vi "CSS grouping with vector space.vi"() -> ()   [LabVIEW 2014]
uses:
  <vilib>/Utility/file.llb/Read From Spreadsheet File (string).vi
  <vilib>/Utility/file.llb/Write To Spreadsheet File (string).vi
panel:
  in  "file path (to write) 2":path
  in  "save":bool
  in  "cycles":i32=1
  out "Array 4":string[](array[string])
  in  "cluster centers (original) 7":string[](array[string])=["0 -1 1 -4 0", "0 -1 2 -2 0", "0 -2 3 -3 0", "0 -3 4 -4 0", "0 -1 1 -4 4 -3 0", "0 -1 2 -2 3 -3 0", "0 -4 1 -1 2 -2 0", "0 -4 4 -3 3 -2 0", "0 -1 1 -4 0 -2 3 -3 0", "0 -1 2 -2 0 -4 4 -3 0"]
  out "vector positions only":dbl[][](array[numeric])
  out "Array 3":dbl[][](array[numeric])
  out "Array 2":dbl[][](array[numeric])
  out "Array":dbl[][](array[numeric])
  out "Assignment (enhanced)":string[](array[string])
  out "Assignment":string[](array[string])
  out "all rows":string[][](array[string])
  in  "cluster centers (original) 5":string[](array[string])=["0 -1 1 -4 0 -4 1 -1 0 -1 1 -4 0 -4 1 -1 0 -1 1 -4 0 -4 1 -1 0 -1 0 -1 1 -4 0 -4 1 -1 0", "0 -1 2 -2 0 -2 2 -1 0 -1 2 -2 0 -2 2 -1 0 -1 2 -2 0 -2 2 -1 0 -1 0 -1 2 -2 0 -2 2 -1 0", "0 -2 3 -3 0 -3 3 -2 0 -2 3 -3 0 -3 3 -2 0 -2 3 -3 0 -3 3 -2 0 -2 0 -2 3 -3 0 -3 3 -2 0", "0 -3 4 -4 0 -4 4 -3 0 -3 4 -4 0 -4 4 -3 0 -3 4 -4 0 -4 4 -3 0 -3 0 -3 4 -4 0 -4 4 -3 0", "0 -1 1 -4 4 -3 0 -3 4 -4 1 -1 0 -1 1 -4 4 -3 0 -3 4 -4 1 -1 0 -1 1 -4 4 -3 0 -3 4 -4 1 -1 0 -1 1 -4 4 -3 0 -3 4 -4 1 -1 0", "0 -1 2 -2 3 -3 0 -3 3 -2 2 -1 0 -1 2 -2 3 -3 0 -3 3 -2 2 -1 0 -1 2 -2 3 -3 0 -3 3 -2 2 -1 0 -1 2 -2 3 -3 0 -3 3 -2 2 -1 0", "0 -4 1 -1 2 -2 0 -2 2 -1 1 -4 0 -4 1 -1 2 -2 0 -2 2 -1 1 -4 0 -4 1 -1 2 -2 0 -2 2 -1 1 -4 0 -4 1 -1 2 -2 0 -2 2 -1 1 -4 0", "0 -4 4 -3 3 -2 0 -2 3 -3 4 -4 0 -4 4 -3 3 -2 0 -2 3 -3 4 -4 0 -4 4 -3 3 -2 0 -2 3 -3 4 -4 0 -4 4 -3 3 -2 0 -2 3 -3 4 -4 0", "0 -1 1 -4 0 -2 3 -3 0 -3 3 -2 0 -4 1 -1 0 -1 1 -4 0 -2 3 -3 0 -3 3 -2 0 -4 1 -1 0 -1 1 -4 0 -2 3 -3 0 -3 3 -2 0 -4 1 -1 0 -1 1 -4 0 -2 3 -3 0 -3 3 -2 0 -4 1 -1 0", "0 -1 2 -2 0 -4 4 -3 0 -3 4 -4 0 -2 2 -1 0 -1 2 -2 0 -4 4 -3 0 -3 4 -4 0 -2 2 -1 0 -1 2 -2 0 -4 4 -3 0 -3 4 -4 0 -2 2 -1 0 -1 2 -2 0 -4 4 -3 0 -3 4 -4 0 -2 2 -1 0"]
  in  "cluster centers (original) 4":string[](array[string])=["0 -1 1 -4 0 -4 1 -1 0 -1 1 -4 0 -4 1 -1 0", "0 -1 2 -2 0 -2 2 -1 0 -1 2 -2 0 -2 2 -1 0", "0 -2 3 -3 0 -3 3 -2 0 -2 3 -3 0 -3 3 -2 0", "0 -3 4 -4 0 -4 4 -3 0 -3 4 -4 0 -4 4 -3 0", "0 -1 1 -4 4 -3 0 -3 4 -4 1 -1 0 -1 1 -4 4 -3 0 -3 4 -4 1 -1 0", "0 -1 2 -2 3 -3 0 -3 3 -2 2 -1 0 -1 2 -2 3 -3 0 -3 3 -2 2 -1 0", "0 -4 1 -1 2 -2 0 -2 2 -1 1 -4 0 -4 1 -1 2 -2 0 -2 2 -1 1 -4 0", "0 -4 4 -3 3 -2 0 -2 3 -3 4 -4 0 -4 4 -3 3 -2 0 -2 3 -3 4 -4 0", "0 -1 1 -4 0 -2 3 -3 0 -3 3 -2 0 -4 1 -1 0 -1 1 -4 0 -2 3 -3 0 -3 3 -2 0 -4 1 -1 0", "0 -1 2 -2 0 -4 4 -3 0 -3 4 -4 0 -2 2 -1 0 -1 2 -2 0 -4 4 -3 0 -3 4 -4 0 -2 2 -1 0"]
  out "size(s)":i32
  in  "cluster centers (original) 3":string[](array[string])=["0 -1 1 -4 0 -4 1 -1 0 -1 1 -4 0 -4 1 -1 0 -1 1 -4 0 -4 1 -1 0", "0 -1 2 -2 0 -2 2 -1 0 -1 2 -2 0 -2 2 -1 0 -1 2 -2 0 -2 2 -1 0", "0 -2 3 -3 0 -3 3 -2 0 -2 3 -3 0 -3 3 -2 0 -2 3 -3 0 -3 3 -2 0", "0 -3 4 -4 0 -4 4 -3 0 -3 4 -4 0 -4 4 -3 0 -3 4 -4 0 -4 4 -3 0", "0 -1 1 -4 4 -3 0 -3 4 -4 1 -1 0 -1 1 -4 4 -3 0 -3 4 -4 1 -1 0 -1 1 -4 4 -3 0 -3 4 -4 1 -1 0", "0 -1 2 -2 3 -3 0 -3 3 -2 2 -1 0 -1 2 -2 3 -3 0 -3 3 -2 2 -1 0 -1 2 -2 3 -3 0 -3 3 -2 2 -1 0", "0 -4 1 -1 2 -2 0 -2 2 -1 1 -4 0 -4 1 -1 2 -2 0 -2 2 -1 1 -4 0 -4 1 -1 2 -2 0 -2 2 -1 1 -4 0", "0 -4 4 -3 3 -2 0 -2 3 -3 4 -4 0 -4 4 -3 3 -2 0 -2 3 -3 4 -4 0 -4 4 -3 3 -2 0 -2 3 -3 4 -4 0", "0 -1 1 -4 0 -2 3 -3 0 -3 3 -2 0 -4 1 -1 0 -1 1 -4 0 -2 3 -3 0 -3 3 -2 0 -4 1 -1 0 -1 1 -4 0 -2 3 -3 0 -3 3 -2 0 -4 1 -1 0", "0 -1 2 -2 0 -4 4 -3 0 -3 4 -4 0 -2 2 -1 0 -1 2 -2 0 -4 4 -3 0 -3 4 -4 0 -2 2 -1 0 -1 2 -2 0 -4 4 -3 0 -3 4 -4 0 -2 2 -1 0"]
  in  "cluster centers (original) 2":string[](array[string])=["0 -1 1 -4 0 -4 1 -1 0", "0 -1 2 -2 0 -2 2 -1 0", "0 -2 3 -3 0 -3 3 -2 0", "0 -3 4 -4 0 -4 4 -3 0", "0 -1 1 -4 4 -3 0 -3 4 -4 1 -1 0", "0 -1 2 -2 3 -3 0 -3 3 -2 2 -1 0", "0 -4 1 -1 2 -2 0 -2 2 -1 1 -4 0", "0 -4 4 -3 3 -2 0 -2 3 -3 4 -4 0", "0 -1 1 -4 0 -2 3 -3 0 -3 3 -2 0 -4 1 -1 0", "0 -1 2 -2 0 -4 4 -3 0 -3 4 -4 0 -2 2 -1 0"]
  out "accuracy":string[][](array[string])
  in  "cluster centers (original) long 5":string[](array[string])=["1 0 -1 1 -1 0 -4 1 -4 0 1 0 -1 1 -1 0 -4 1 -4 0 1 0 -1 1 -1 0 -4 1 -4 0 1 0 -1 1 -1 0 -4 1 -4 0 1 0 -1 1 -1 0 -4 1 -4 0 1", "2 0 -1 2 -1 0 -2 2 -2 0 2 0 -1 2 -1 0 -2 2 -2 0 2 0 -1 2 -1 0 -2 2 -2 0 2 0 -1 2 -1 0 -2 2 -2 0 2 0 -1 2 -1 0 -2 2 -2 0 2", "3 0 -3 3 -3 0 -2 3 -2 0 3 0 -3 3 -3 0 -2 3 -2 0 3 0 -3 3 -3 0 -2 3 -2 0 3 0 -3 3 -3 0 -2 3 -2 0 3 0 -3 3 -3 0 -2 3 -2 0 3", "4 0 -3 4 -3 0 -4 4 -4 0 4 0 -3 4 -3 0 -4 4 -4 0 4 0 -3 4 -3 0 -4 4 -4 0 4 0 -3 4 -3 0 -4 4 -4 0 4 0 -3 4 -3 0 -4 4 -4 0 4", "-1 1 -4 0 -4 4 -3 4 -4 0 -4 1 -1 1 -4 0 -4 4 -3 4 -4 0 -4 1 -1 1 -4 0 -4 4 -3 4 -4 0 -4 1 -1 1 -4 0 -4 4 -3 4 -4 0 -4 1 -1 1 -4 0 -4 4 -3 4 -4 0 -4 1 -1", "-1 2 -2 0 -2 3 -3 3 -2 0 -2 2 -1 2 -2 0 -2 3 -3 3 -2 0 -2 2 -1 2 -2 0 -2 3 -3 3 -2 0 -2 2 -1 2 -2 0 -2 3 -3 3 -2 0 -2 2 -1 2 -2 0 -2 3 -3 3 -2 0 -2 2 -1", "-4 1 -1 0 -1 2 -2 2 -1 0 -1 1 -4 1 -1 0 -1 2 -2 2 -1 0 -1 1 -4 1 -1 0 -1 2 -2 2 -1 0 -1 1 -4 1 -1 0 -1 2 -2 2 -1 0 -1 1 -4 1 -1 0 -1 2 -2 2 -1 0 -1 1 -4", "-4 4 -3 0 -3 3 -2 3 -3 0 -3 4 -4 4 -3 0 -3 3 -2 3 -3 0 -3 4 -4 4 -3 0 -3 3 -2 3 -3 0 -3 4 -4 4 -3 0 -3 3 -2 3 -3 0 -3 4 -4 4 -3 0 -3 3 -2 3 -3 0 -3 4 -4", "0 -4 1 -1 0 -3 3 -2 3 -3 0 -1 1 -4 0 -4 1 -1 0 -3 3 -2 3 -3 0 -1 1 -4 0 -4 1 -1 0 -3 3 -2 3 -3 0 -1 1 -4 0 -4 1 -1 0 -3 3 -2 3 -3 0 -1 1 -4 0 -4 1 -1 0 -3 3 -2 3 -3 0 -1 1 -4 0", "0 -4 4 -3 0 -1 2 -2 2 -1 0 -3 4 -4 0 -4 4 -3 0 -1 2 -2 2 -1 0 -3 4 -4 0 -4 4 -3 0 -1 2 -2 2 -1 0 -3 4 -4 0 -4 4 -3 0 -1 2 -2 2 -1 0 -3 4 -4 0 -4 4 -3 0 -1 2 -2 2 -1 0 -3 4 -4 0"]
  in  "cluster centers (original) long 4":string[](array[string])=["1 0 -1 1 -1 0 -4 1 -4 0 1 0 -1 1 -1 0 -4 1 -4 0 1 0 -1 1 -1 0 -4 1 -4 0 1 0 -1 1 -1 0 -4 1 -4 0 1", "2 0 -1 2 -1 0 -2 2 -2 0 2 0 -1 2 -1 0 -2 2 -2 0 2 0 -1 2 -1 0 -2 2 -2 0 2 0 -1 2 -1 0 -2 2 -2 0 2", "3 0 -3 3 -3 0 -2 3 -2 0 3 0 -3 3 -3 0 -2 3 -2 0 3 0 -3 3 -3 0 -2 3 -2 0 3 0 -3 3 -3 0 -2 3 -2 0 3", "4 0 -3 4 -3 0 -4 4 -4 0 4 0 -3 4 -3 0 -4 4 -4 0 4 0 -3 4 -3 0 -4 4 -4 0 4 0 -3 4 -3 0 -4 4 -4 0 4", "-1 1 -4 0 -4 4 -3 4 -4 0 -4 1 -1 1 -4 0 -4 4 -3 4 -4 0 -4 1 -1 1 -4 0 -4 4 -3 4 -4 0 -4 1 -1 1 -4 0 -4 4 -3 4 -4 0 -4 1 -1", "-1 2 -2 0 -2 3 -3 3 -2 0 -2 2 -1 2 -2 0 -2 3 -3 3 -2 0 -2 2 -1 2 -2 0 -2 3 -3 3 -2 0 -2 2 -1 2 -2 0 -2 3 -3 3 -2 0 -2 2 -1", "-4 1 -1 0 -1 2 -2 2 -1 0 -1 1 -4 1 -1 0 -1 2 -2 2 -1 0 -1 1 -4 1 -1 0 -1 2 -2 2 -1 0 -1 1 -4 1 -1 0 -1 2 -2 2 -1 0 -1 1 -4", "-4 4 -3 0 -3 3 -2 3 -3 0 -3 4 -4 4 -3 0 -3 3 -2 3 -3 0 -3 4 -4 4 -3 0 -3 3 -2 3 -3 0 -3 4 -4 4 -3 0 -3 3 -2 3 -3 0 -3 4 -4", "0 -4 1 -1 0 -3 3 -2 3 -3 0 -1 1 -4 0 -4 1 -1 0 -3 3 -2 3 -3 0 -1 1 -4 0 -4 1 -1 0 -3 3 -2 3 -3 0 -1 1 -4 0 -4 1 -1 0 -3 3 -2 3 -3 0 -1 1 -4 0", "0 -4 4 -3 0 -1 2 -2 2 -1 0 -3 4 -4 0 -4 4 -3 0 -1 2 -2 2 -1 0 -3 4 -4 0 -4 4 -3 0 -1 2 -2 2 -1 0 -3 4 -4 0 -4 4 -3 0 -1 2 -2 2 -1 0 -3 4 -4 0"]
  in  "cluster centers (original) long 3":string[](array[string])=["1 0 -1 1 -1 0 -4 1 -4 0 1 0 -1 1 -1 0 -4 1 -4 0 1 0 -1 1 -1 0 -4 1 -4 0 1", "2 0 -1 2 -1 0 -2 2 -2 0 2 0 -1 2 -1 0 -2 2 -2 0 2 0 -1 2 -1 0 -2 2 -2 0 2", "3 0 -3 3 -3 0 -2 3 -2 0 3 0 -3 3 -3 0 -2 3 -2 0 3 0 -3 3 -3 0 -2 3 -2 0 3", "4 0 -3 4 -3 0 -4 4 -4 0 4 0 -3 4 -3 0 -4 4 -4 0 4 0 -3 4 -3 0 -4 4 -4 0 4", "-1 1 -4 0 -4 4 -3 4 -4 0 -4 1 -1 1 -4 0 -4 4 -3 4 -4 0 -4 1 -1 1 -4 0 -4 4 -3 4 -4 0 -4 1 -1", "-1 2 -2 0 -2 3 -3 3 -2 0 -2 2 -1 2 -2 0 -2 3 -3 3 -2 0 -2 2 -1 2 -2 0 -2 3 -3 3 -2 0 -2 2 -1", "-4 1 -1 0 -1 2 -2 2 -1 0 -1 1 -4 1 -1 0 -1 2 -2 2 -1 0 -1 1 -4 1 -1 0 -1 2 -2 2 -1 0 -1 1 -4", "-4 4 -3 0 -3 3 -2 3 -3 0 -3 4 -4 4 -3 0 -3 3 -2 3 -3 0 -3 4 -4 4 -3 0 -3 3 -2 3 -3 0 -3 4 -4", "0 -4 1 -1 0 -3 3 -2 3 -3 0 -1 1 -4 0 -4 1 -1 0 -3 3 -2 3 -3 0 -1 1 -4 0 -4 1 -1 0 -3 3 -2 3 -3 0 -1 1 -4 0", "0 -4 4 -3 0 -1 2 -2 2 -1 0 -3 4 -4 0 -4 4 -3 0 -1 2 -2 2 -1 0 -3 4 -4 0 -4 4 -3 0 -1 2 -2 2 -1 0 -3 4 -4 0"]
  in  "cluster centers (original) long":string[](array[string])=["1 0 -1 1 -1 0 -4 1 -4 0 1 0 -1 1 -1 0 -4 1 -4 0 1", "2 0 -1 2 -1 0 -2 2 -2 0 2 0 -1 2 -1 0 -2 2 -2 0 2", "3 0 -3 3 -3 0 -2 3 -2 0 3 0 -3 3 -3 0 -2 3 -2 0 3", "4 0 -3 4 -3 0 -4 4 -4 0 4 0 -3 4 -3 0 -4 4 -4 0 4", "-1 1 -4 0 -4 4 -3 4 -4 0 -4 1 -1 1 -4 0 -4 4 -3 4 -4 0 -4 1 -1", "-1 2 -2 0 -2 3 -3 3 -2 0 -2 2 -1 2 -2 0 -2 3 -3 3 -2 0 -2 2 -1", "-4 1 -1 0 -1 2 -2 2 -1 0 -1 1 -4 1 -1 0 -1 2 -2 2 -1 0 -1 1 -4", "-4 4 -3 0 -3 3 -2 3 -3 0 -3 4 -4 4 -3 0 -3 3 -2 3 -3 0 -3 4 -4", "0 -4 1 -1 0 -3 3 -2 3 -3 0 -1 1 -4 0 -4 1 -1 0 -3 3 -2 3 -3 0 -1 1 -4 0", "0 -4 4 -3 0 -1 2 -2 2 -1 0 -3 4 -4 0 -4 4 -3 0 -1 2 -2 2 -1 0 -3 4 -4 0"]
  out "Results":string[][](array[string])
  in  "file path (dialog if empty)":path=path "K:/PhD work/PhD research work 2/Common substring validation/documentation/Data final results/Common substrings (ground truth 2 CHECKED).txt"
  in  "cluster centers (original)":string[](array[string])=["1 0 -1 1 -1 0 -4 1 -4 0 1", "2 0 -1 2 -1 0 -2 2 -2 0 2", "3 0 -3 3 -3 0 -2 3 -2 0 3", "4 0 -3 4 -3 0 -4 4 -4 0 4", "-1 1 -4 0 -4 4 -3 4 -4 0 -4 1 -1", "-1 2 -2 0 -2 3 -3 3 -2 0 -2 2 -1", "-4 1 -1 0 -1 2 -2 2 -1 0 -1 1 -4", "-4 4 -3 0 -3 3 -2 3 -3 0 -3 4 -4", "0 -4 1 -1 0 -3 3 -2 3 -3 0 -1 1 -4 0", "0 -4 4 -3 0 -1 2 -2 2 -1 0 -3 4 -4 0"]
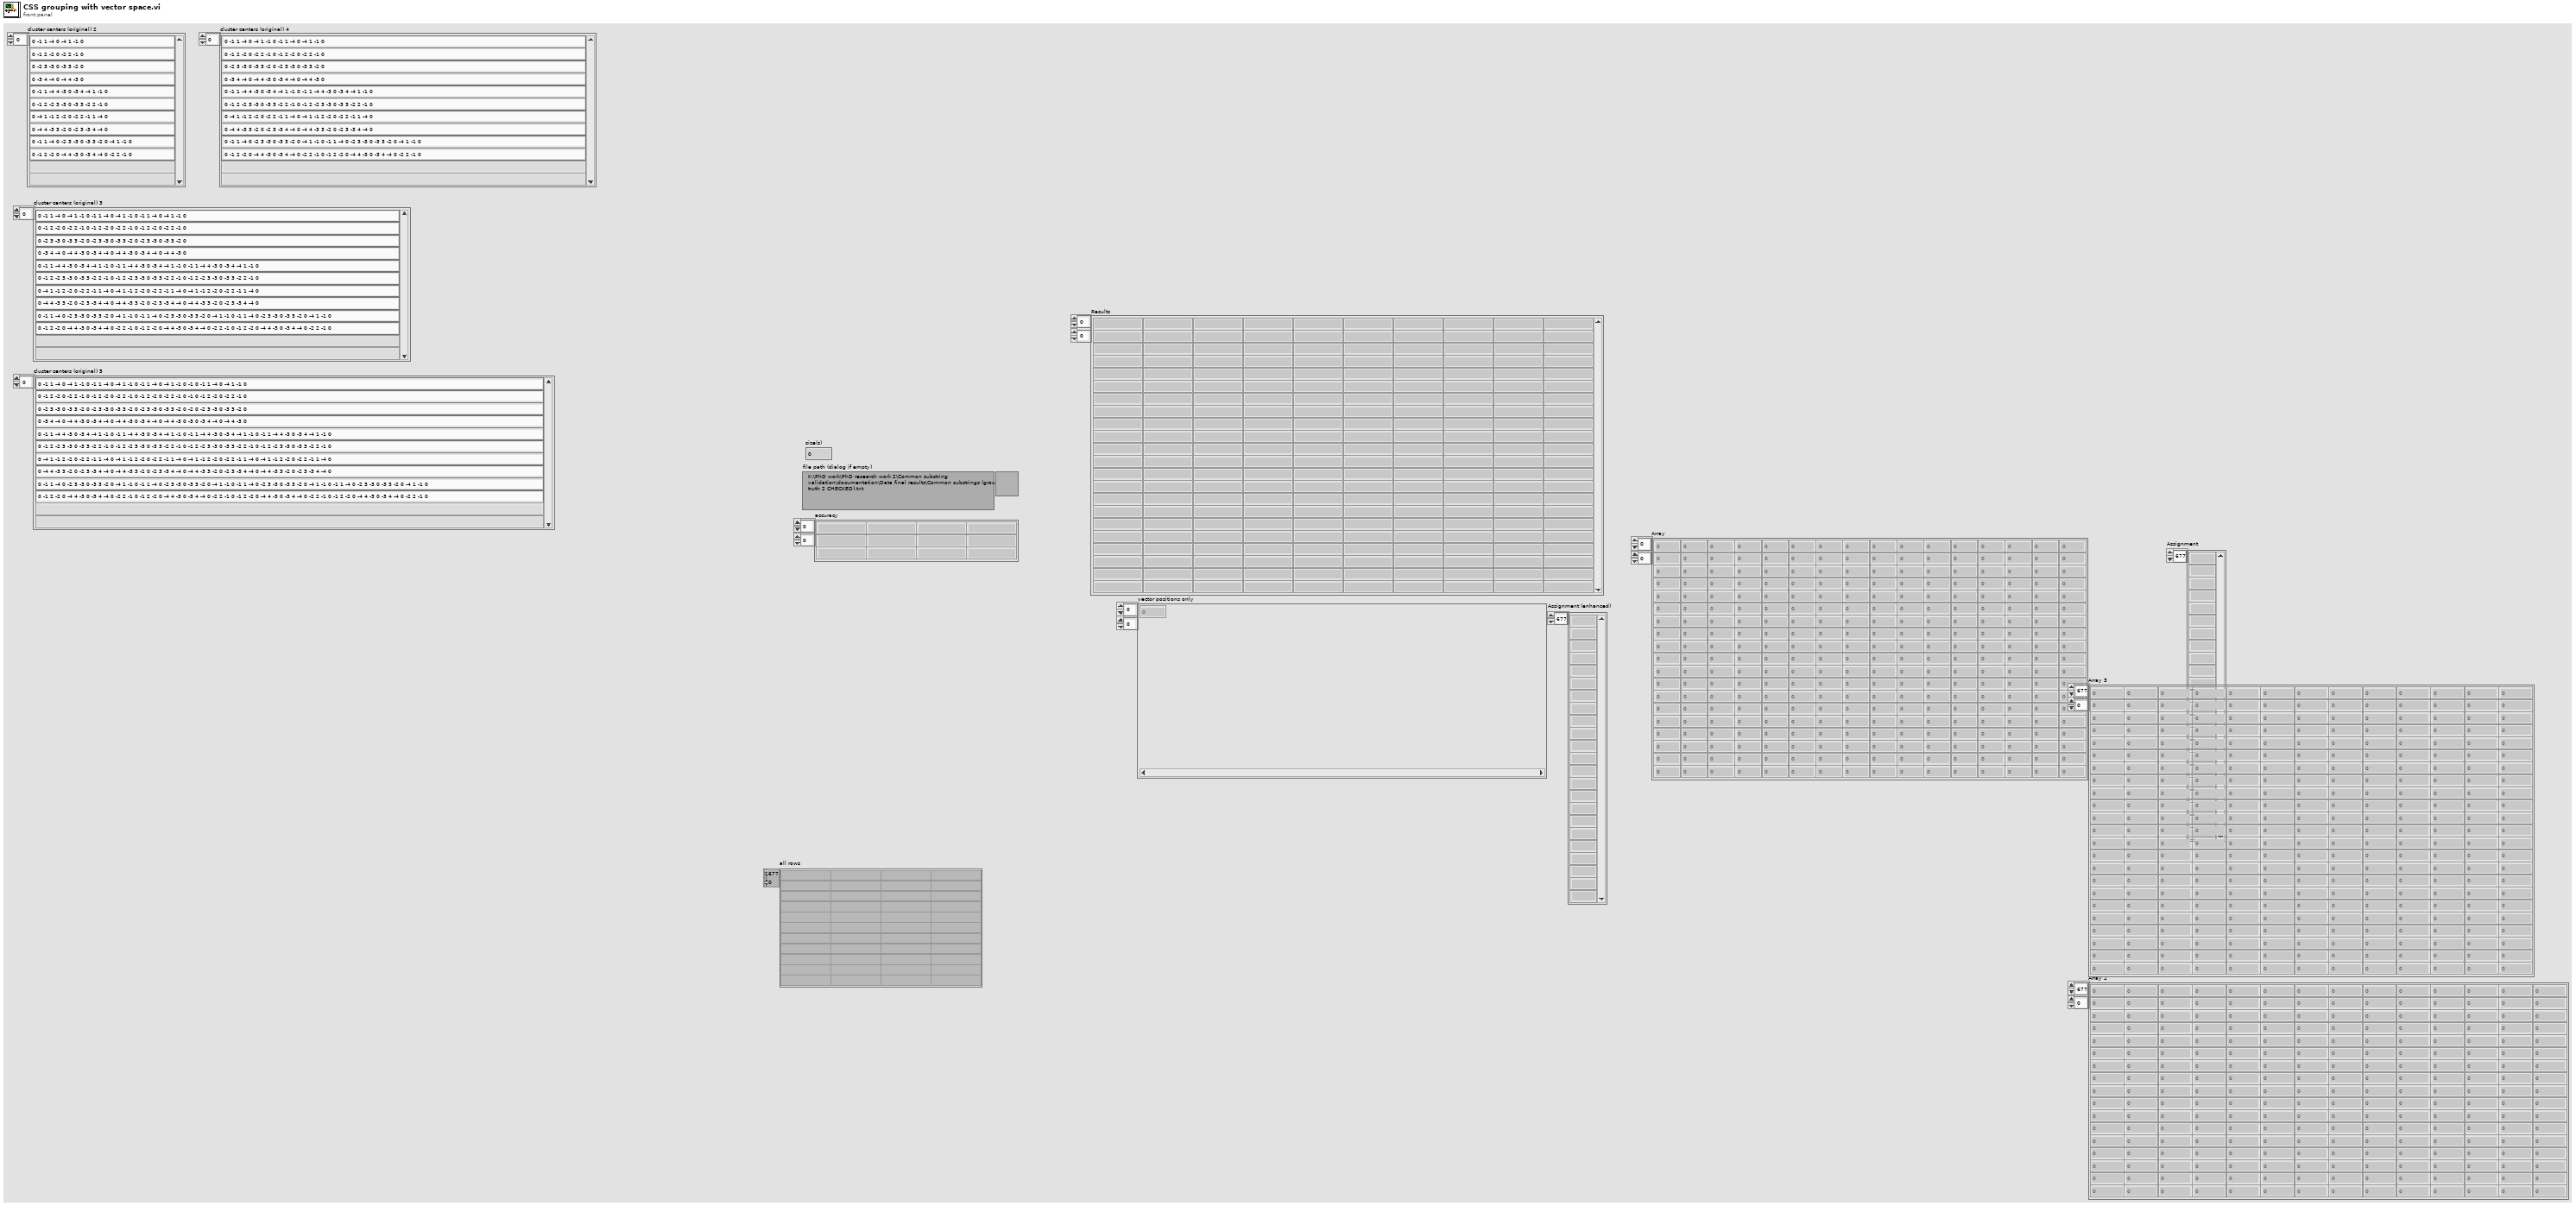
[diagram p1: front panel]
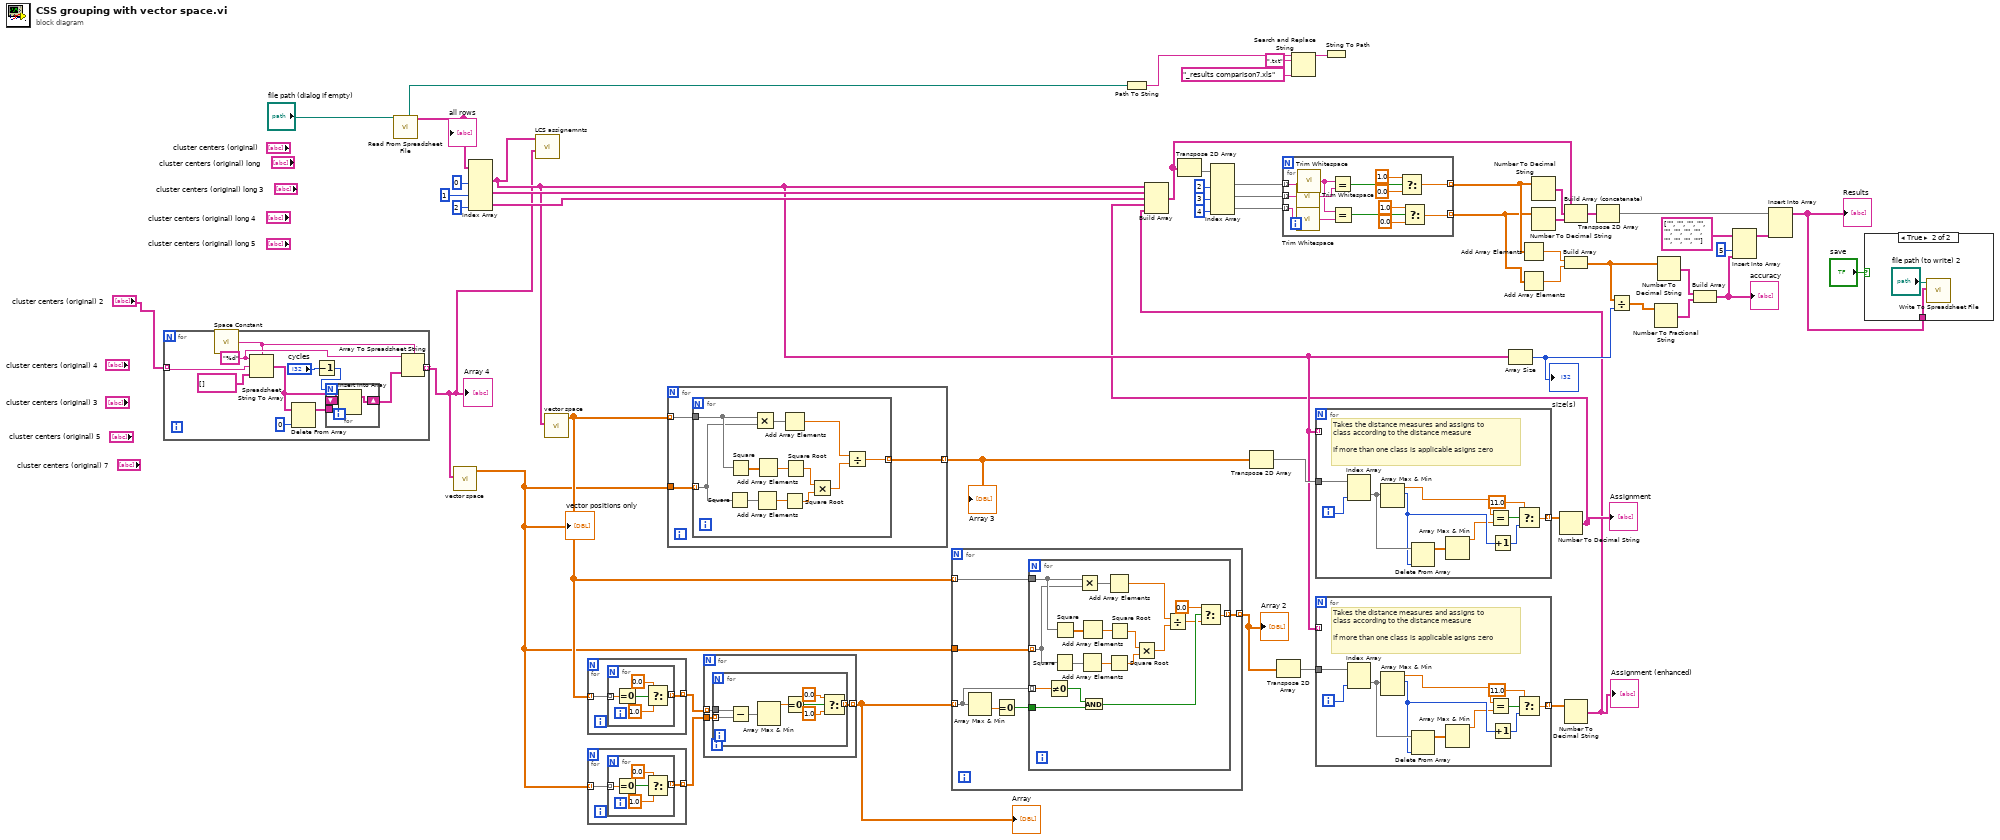
[diagram p0: block diagram]
diagram:
  n1 = for {
    tunnel: [w62] -> w4 mode=indexing
    tunnel: "cluster centers (original) 2" -> [w58] mode=indexing
    w63 = "%d" ("format string")
    n2 = call <vilib>:"Space Constant.vi"() -> ("String"=w61:string)
    n3 = Spreadsheet String To Array(delimiter (Tab)=w61, format string=w63, spreadsheet string=w58, array type (2D Dbl)=string[] []) -> (array=w57:string[])
    n4 = Delete From Array(array=w57, index=0) -> (array with subset deleted=w56:string[])  [unwired: 1 in, 1 out]
    n5 = Decrement(x="cycles") -> (x-1=w60:i32)
    n6 = for {
      N: w60 -> [_]
      tunnel: w56 -> [w68]
      shift-right: [w67] -> w64
      shift-left: w57 -> [w69]
      n7 = Insert Into Array(array=w69, new element=w68) -> (w67:string[])  [unwired: 1 in]
    }
    n8 = Array To Spreadsheet String(delimiter (Tab)=w61, array=w64, 3:w63) -> (spreadsheet string=w62:string)
  }
  "Array 4" <- w4
  n9 = call-poly <vilib>:"Read From Spreadsheet File.vi"("file path (dialog if empty)"="file path (dialog if empty)") -> ("all rows"=w21:string[][], "new file path (Not A Path if cancelled)"=w53:path)  [unwired: 6 in, 3 out]
  "all rows" <- w21
  n10 = call "vector space.vi"("Full transition sequence from service to end"=w4) -> ("vector positions only"=w5:dbl[][])  [unwired: 8 in, 2 out]
  "vector positions only" <- w5
  n11 = Index Array(array=w21, index (col) #1=0 ("disabled index (col)"), index (col) #2=1 ("index (col)"), index (col) #3=2 ("index (col)")) -> (element #1=w14:string[], element #2=w20:string[], element #3=w19:string[])  [unwired: 3 in]
  n12 = call "LCS assignemnts.vi"("cluster centers"=w4, "Patterns in"=w14) -> ()  [unwired: 1 in, 9 out]
  n13 = call "vector space.vi"("Full transition sequence from service to end"=w14) -> ("vector positions only"=w6:dbl[][])  [unwired: 8 in, 2 out]
  n14 = for {
    tunnel: w6 -> [w71] mode=indexing
    tunnel: [w70] -> w13 mode=indexing
    n15 = for {
      tunnel: w71 -> [w76] mode=indexing
      tunnel: [w72] -> w70 mode=indexing
      n16 = Equal To 0?(x=w76) -> (x = 0?=w75:bool)
      n17 = Select(t=0.0, s=w75, f=1.0 ("t")) -> (s? t:f=w72:dbl)
    }
  }
  n18 = for {
    tunnel: w5 -> [w78] mode=indexing
    tunnel: [w77] -> w11 mode=indexing
    n19 = for {
      tunnel: w78 -> [w83] mode=indexing
      tunnel: [w79] -> w77 mode=indexing
      n20 = Equal To 0?(x=w83) -> (x = 0?=w82:bool)
      n21 = Select(t=0.0, s=w82, f=1.0 ("t")) -> (s? t:f=w79:dbl)
    }
  }
  n22 = for {
    tunnel: w6 -> [w85] mode=indexing
    tunnel: w5 -> [w86]
    tunnel: [w84] -> w9 mode=indexing
    n23 = for {
      tunnel: w86 -> [w88] mode=indexing
      tunnel: w85 -> [w98]
      tunnel: [w87] -> w84 mode=indexing
      n24 = Square(x=w88) -> (x^2=w93:dbl[])
      n25 = Square(x=w98) -> (x^2=w96:dbl[])
      n26 = Multiply(x=w98, y=w88) -> (x*y=w97:dbl[])
      n27 = Add Array Elements(numeric array=w93) -> (sum=w94:dbl)
      n28 = Add Array Elements(numeric array=w96) -> (sum=w95:dbl)
      n29 = Add Array Elements(numeric array=w97) -> (sum=w89:dbl)
      n30 = Square Root(x=w94) -> (sqrt(x)=w91:dbl)
      n31 = Square Root(x=w95) -> (sqrt(x)=w92:dbl)
      n32 = Multiply(x=w92, y=w91) -> (x*y=w90:dbl)
      n33 = Divide(x=w89, y=w90) -> (x/y=w87:dbl)
    }
  }
  "Array 3" <- w9
  n34 = for {
    tunnel: w13 -> [w101] mode=indexing
    tunnel: w11 -> [w100]
    tunnel: [w99] -> w12 mode=indexing
    n35 = for {
      tunnel: w101 -> [w109]
      tunnel: w100 -> [w108] mode=indexing
      tunnel: [w102] -> w99 mode=indexing
      n36 = Subtract(x=w109, y=w108) -> (x-y=w107:dbl[])
      n37 = Array Max & Min(array=w107) -> (max value=w106:dbl)  [unwired: 3 out]
      n38 = Equal To 0?(x=w106) -> (x = 0?=w105:bool)
      n39 = Select(t=0.0, s=w105, f=1.0) -> (s? t:f=w102:dbl)
    }
  }
  "Array" <- w12
  n40 = for {
    tunnel: w6 -> [w114] mode=indexing
    tunnel: w5 -> [w115]
    tunnel: [w113] -> w10 mode=indexing
    tunnel: w12 -> [w110] mode=indexing
    n41 = Array Max & Min(array=w110) -> (min value=w112:dbl)  [unwired: 3 out]
    n42 = Equal To 0?(x=w112) -> (x = 0?=w111:bool)
    n43 = for {
      tunnel: w115 -> [w127] mode=indexing
      tunnel: w114 -> [w133]
      tunnel: [w116] -> w113 mode=indexing
      tunnel: w111 -> [w120]
      tunnel: w110 -> [w122] mode=indexing
      n44 = Not Equal To 0?(x=w122) -> (x != 0?=w121:bool)
      n45 = Square(x=w127) -> (x^2=w128:dbl[])
      n46 = Square(x=w133) -> (x^2=w131:dbl[])
      n47 = Multiply(x=w133, y=w127) -> (x*y=w132:dbl[])
      n48 = Add Array Elements(numeric array=w128) -> (sum=w129:dbl)
      n49 = Add Array Elements(numeric array=w131) -> (sum=w130:dbl)
      n50 = And(x=w121, y=w120) -> (x .and. y?=w119:bool)
      n51 = Add Array Elements(numeric array=w132) -> (sum=w123:dbl)
      n52 = Square Root(x=w129) -> (sqrt(x)=w125:dbl)
      n53 = Square Root(x=w130) -> (sqrt(x)=w126:dbl)
      n54 = Multiply(x=w126, y=w125) -> (x*y=w124:dbl)
      n55 = Divide(x=w123, y=w124) -> (x/y=w117:dbl)
      n56 = Select(t=0.0, s=w119, f=w117) -> (s? t:f=w116:dbl)
    }
  }
  "Array 2" <- w10
  n57 = Path To String(path=w53) -> (string=w52:string)
  n58 = Transpose 2D Array(2D array=w9) -> (transposed array=w17:dbl[][])
  n59 = Transpose 2D Array(2D array=w10) -> (transposed array=w15:dbl[][])
  n60 = Search and Replace String(input string=w52, search string=".txt", replace string="_results comparison7.xls" ("replace string (\"\")")) -> (result string=w49:string)  [unwired: 5 in, 3 out]
  n61 = for {
    tunnel: w17 -> [w144]
    tunnel: [w134] -> w18 mode=indexing
    tunnel: w14 -> [_] mode=indexing
    i -> [w143]
    # "Takes the distance measures and assigns to \nclass according to the distance measure\n\nIf more than one class is applicable asigns zero"
    n62 = Index Array(array=w144, index (col)=w143) -> (element=w138:dbl[])  [unwired: 1 in]
    n63 = Array Max & Min(array=w138) -> (max value=w137:dbl, max index (indices)=w136:i32)  [unwired: 2 out]
    n64 = Delete From Array(array=w138, index=w136) -> (array with subset deleted=w142:dbl[])  [unwired: 1 in, 1 out]
    n65 = Array Max & Min(array=w142) -> (max value=w135:dbl)  [unwired: 3 out]
    n66 = Equal?(x=w137, y=w135) -> (x = y?=w141:bool)
    n67 = Increment(x=w136) -> (x+1=w139:i32)
    n68 = Select(t=11.0, s=w141, f=w139) -> (s? t:f=w134:dbl)
  }
  n69 = for {
    tunnel: w15 -> [w155]
    tunnel: [w145] -> w16 mode=indexing
    tunnel: w14 -> [_] mode=indexing
    i -> [w154]
    # "Takes the distance measures and assigns to \nclass according to the distance measure\n\nIf more than one class is applicable asigns zero"
    n70 = Index Array(array=w155, index (col)=w154) -> (element=w149:dbl[])  [unwired: 1 in]
    n71 = Array Max & Min(array=w149) -> (max value=w148:dbl, max index (indices)=w147:i32)  [unwired: 2 out]
    n72 = Delete From Array(array=w149, index=w147) -> (array with subset deleted=w153:dbl[])  [unwired: 1 in, 1 out]
    n73 = Array Max & Min(array=w153) -> (max value=w146:dbl)  [unwired: 3 out]
    n74 = Equal?(x=w148, y=w146) -> (x = y?=w152:bool)
    n75 = Increment(x=w147) -> (x+1=w150:i32)
    n76 = Select(t=11.0, s=w152, f=w150) -> (s? t:f=w145:dbl)
  }
  n77 = String To Path(string=w49) -> ()  [unwired: 1 out]
  n78 = Array Size(array=w14) -> (size(s)=w22:i32)
  "size(s)" <- w22
  n79 = Number To Decimal String(number=w18) -> (decimal integer string=w8:string[])  [unwired: 1 in]
  "Assignment" <- w8
  n80 = Number To Decimal String(number=w16) -> (decimal integer string=w7:string[])  [unwired: 1 in]
  "Assignment (enhanced)" <- w7
  n81 = Build Array(w14, w20, w19, w8, w7) -> (w38:string[][])
  n82 = Transpose 2D Array(2D array=w38) -> (transposed array=w41:string[][])
  n83 = Index Array(array=w41, index (col) #1=2 ("disabled index (col)"), index (col) #2=3 ("index (col)"), index (col) #3=4 ("index (col)")) -> (element #1=w44:string[], element #2=w43:string[], element #3=w42:string[])  [unwired: 3 in]
  n84 = for {
    tunnel: w44 -> [w161] mode=indexing
    tunnel: w43 -> [w160] mode=indexing
    tunnel: w42 -> [w159] mode=indexing
    tunnel: [w163] -> w25 mode=indexing
    tunnel: [w162] -> w24 mode=indexing
    n85 = call <vilib>:"Trim Whitespace.vi"("string"=w160) -> ("trimmed string"=w158:string)  [unwired: 1 in]
    n86 = call <vilib>:"Trim Whitespace.vi"("string"=w159) -> ("trimmed string"=w157:string)  [unwired: 1 in]
    n87 = call <vilib>:"Trim Whitespace.vi"("string"=w161) -> ("trimmed string"=w156:string)  [unwired: 1 in]
    n88 = Equal?(x=w156, y=w158) -> (x = y?=w169:bool)
    n89 = Equal?(x=w156, y=w157) -> (x = y?=w164:bool)
    n90 = Select(t=1.0, s=w169, f=0.0) -> (s? t:f=w163:dbl)
    n91 = Select(t=1.0, s=w164, f=0.0) -> (s? t:f=w162:dbl)
  }
  n92 = Add Array Elements(numeric array=w25) -> (sum=w26:dbl)
  n93 = Add Array Elements(numeric array=w24) -> (sum=w27:dbl)
  n94 = Number To Decimal String(number=w25) -> (decimal integer string=w40:string[])  [unwired: 1 in]
  n95 = Number To Decimal String(number=w24) -> (decimal integer string=w39:string[])  [unwired: 1 in]
  n96 = Build Array (concatenate)(w38, w40, w39) -> (w37:string[][])
  n97 = Build Array(w26, w27) -> (w28:dbl[])
  n98 = Transpose 2D Array(2D array=w37) -> (transposed array=w23:string[][])
  n99 = Divide(x=w28, y=w22) -> (x/y=w29:dbl[])
  n100 = Number To Fractional String(number=w29) -> (F-format string=w31:string[])  [unwired: 3 in]
  n101 = Number To Decimal String(number=w28) -> (decimal integer string=w30:string[])  [unwired: 1 in]
  n102 = Build Array(w30, w31) -> (w35:string[][])
  "accuracy" <- w35
  n103 = Insert Into Array(array=string[][] [["", "", "", "", "", ""], ["", "", "", "", "", ""]] ("appended array 3"), index (col)=5 ("disabled index (col)"), new element=w35) -> (w34:string[][])  [unwired: 1 in]
  n104 = Insert Into Array(array=w23, new element=w34) -> (w1:string[][])  [unwired: 2 in]
  "Results" <- w1
  n105 = case shown="True" "save" {
    tunnel: w1 -> [_ w170]
    frame False {
    }
    frame True {
      n106 = call-poly <vilib>:"Write To Spreadsheet File.vi"("2D data"=w170, "file path (dialog if empty)"="file path (to write) 2") -> ()  [unwired: 6 in, 1 out]
    }
  }
